vi "Get Service Descriptor.vi"(8 "error in":errorcluster) -> (0 "error out":errorcluster, 3 "service descriptor":T1)   [LabVIEW 2024, in "Averaged - Broadband.lvlib"]
uses:
  Averaged - Broadband.lvlib
  <vilib>/Plug-In SDKs/Measurements/Helpers/TypeDefs/Service Descriptor.ctl
  <vilib>/Plug-In SDKs/Measurements/Helpers/TypeDefs/Measurement Details.ctl
  <vilib>/Plug-In SDKs/Measurements/Helpers/TypeDefs/Measurement Annotation.ctl
  <vilib>/Plug-In SDKs/Measurements/NI Measurement Plug-In SDK.lvlib
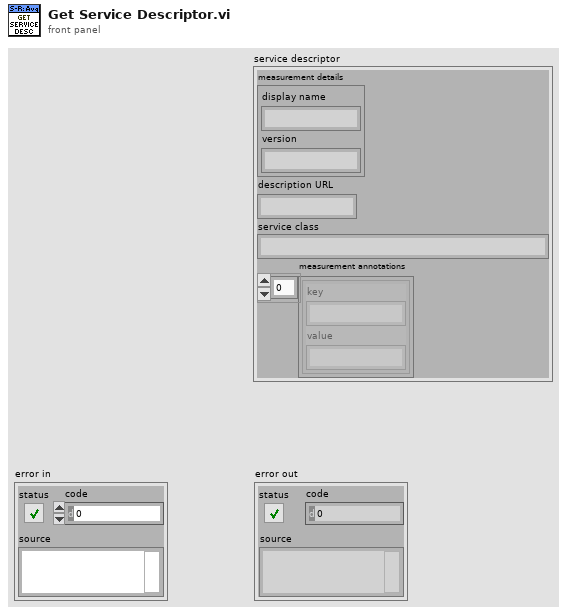
[diagram p1: front panel]
types:
  T1 = typedef "NI Measurement Plug-In SDK.lvlib/Service Descriptor.ctl" = cluster{"measurement details":T2, "description URL":string, "service class":string, "measurement annotations":T3[]}
  T2 = typedef "NI Measurement Plug-In SDK.lvlib/Measurement Details.ctl" = cluster{"display name":string, "version":string}
  T3 = typedef "NI Measurement Plug-In SDK.lvlib/Measurement Annotation.ctl" = cluster{"key":string, "value":string}
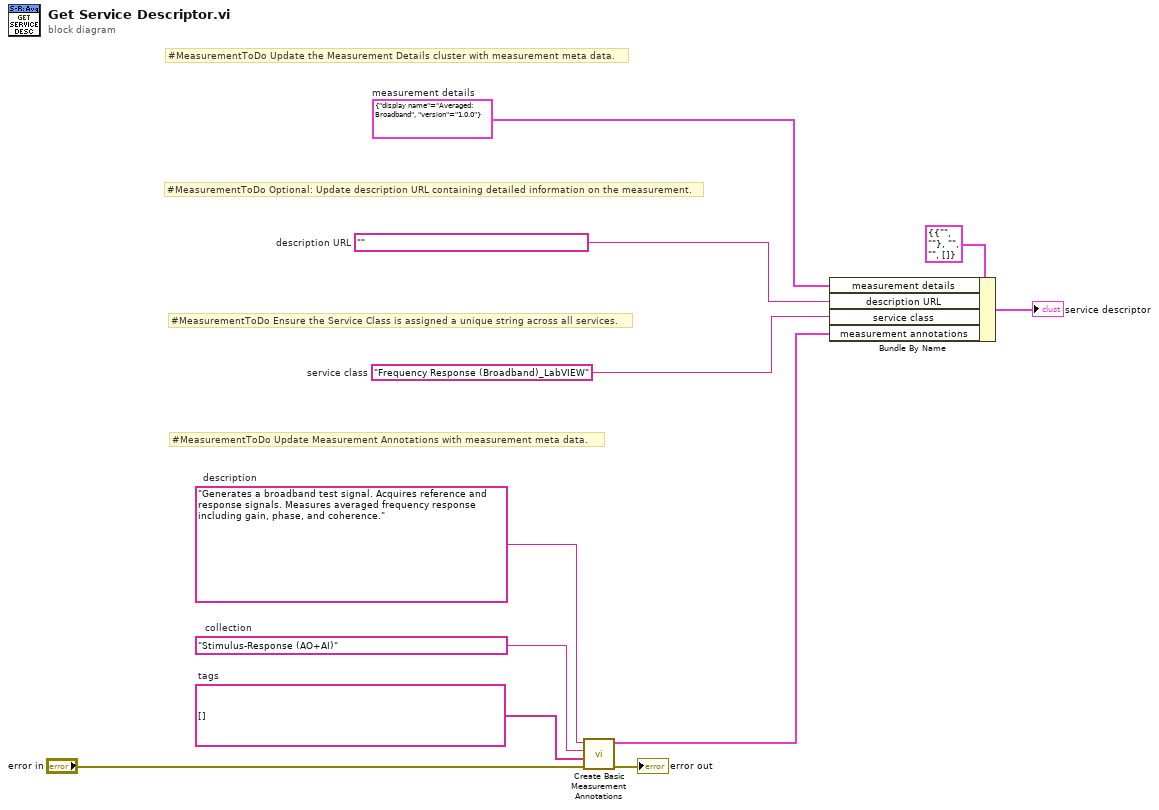
[diagram p0: block diagram]
diagram:
  w5 = ""  # description URL
  w7 = string[] []  # tags
  w8 = "Stimulus-Response (AO+AI)"  # collection
  w9 = "Generates a broadband test signal. Acquires reference and response signals. Measures averaged frequency response including gain, phase, and coherence."  # description
  w6 = T2 {"display name"="Averaged: Broadband", "version"="1.0.0"}  # measurement details
  w4 = "Frequency Response (Broadband)_LabVIEW"  # service class
  # "#MeasurementToDo Optional: Update description URL containing detailed information on the measurement."
  # "#MeasurementToDo Update Measurement Annotations with measurement meta data."
  # "#MeasurementToDo Ensure the Service Class is assigned a unique string across all services."
  # "#MeasurementToDo Update the Measurement Details cluster with measurement meta data."
  n1 = call <vilib>:"Create Basic Measurement Annotations.vi"("error in"="error in", "tags"=w7, "collection"=w8, "description"=w9) -> ("error out"=→"error out":errorcluster, "measurement annotations"=w3:T3[])  [unwired: 6 in]
  n2 = Bundle By Name(cluster=T1 {"measurement details"={"display name"="", "version"=""}, "description URL"="", "service class"="", "measurement annotations"=[]} ("service descriptor"), "measurement details"=w6, "description URL"=w5, "service class"=w4, "measurement annotations"=w3) -> (→"service descriptor":T1)
